vi "Event handler-Averages ValChange.vi"(11 "Averages.NewVal":u16) -> ()   [LabVIEW 2017]
uses:
  Global Variables/gl_UI Parameters.vi
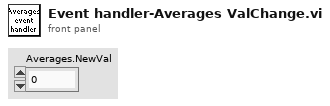
[diagram p1: front panel]
types:
  T1 = cluster{"Z Start":dbl, "Z Stop":dbl, "Z Step":dbl, "Pockels\n@Z Start":u8, "Pockels\n@Z Stop":u8, "# Planes":u16, "Dwell\nTime":sgl, "Zoom":i8, "# Averaged Frames":u16, "PMT 2":i16, "PMT 1":i16, "Laser":u8, "AOL Z":sgl, "Objective":string, "Frame Size":u16, "AOL Mode":u16, "Field of View":u16}
  T2 = typedef "AOL_Globals.ctl" = cluster{"Imaging Protocol":T3, "Number of POI":u16, "Number of Miniscans":u16, "Number of Trials":u16, "Number of Cycles ":u64, "# Averaged Frames":u16, "Laser power (%)":u8, "Pockels":dbl, "Acquisition Length (sec)":dbl, "Fill time (us)":dbl, "POI Dwell time (us)":dbl, "Miniscan Dwell time per pixel (us)":dbl, "PMT 1":dbl, "PMT 2":dbl, "Back Apperture":dbl, "Frame Size":T4, "Center Frequency":dbl, "Field of View":dbl, "DwellTime (us)":dbl, "Wavelength (nm)":dbl, "Zoom":dbl, "AOL Z":dbl, "AOL Mode":T5, "GridXY":dbl, "GridZ":dbl, "TriggerPeriod (sec)":dbl, "Number of Pixels in Miniscan":u16, "Experiment folder path":path, "X centre":dbl, "Y centre":dbl, "Angle (degrees)":dbl, "Plane Mode":T6, "Threshold":u16[], "Regenerate Chirps":bool, "Rectangle ROI length (pixels)":u16, "Rectangle ROI height (pixels)":u16, "AOD fill":u16, "StartupDelay":i32, "Samples Wait after Trigger":u16, "Slip Cycle":u32, "Add Cycle":bool}
  T3 = typedef "Imaging Protocols enum.ctl" = enum16{"AOL Z-Stack", "Motor Z Stack", "Functional Acquisition", "Single Plane Acquisition", "Volume Acquisition", "Live Imaging", "Live Plane Imaging", "Live Volume Imaging"}
  T4 = typedef "Frame Size.ctl" = u16
  T5 = typedef "AOL modes.ctl" = enum16{"Raster", "Structural", "Pointing", "Mini Scan", "Alignment"}
  T6 = typedef "Plane Mode.ctl" = u16
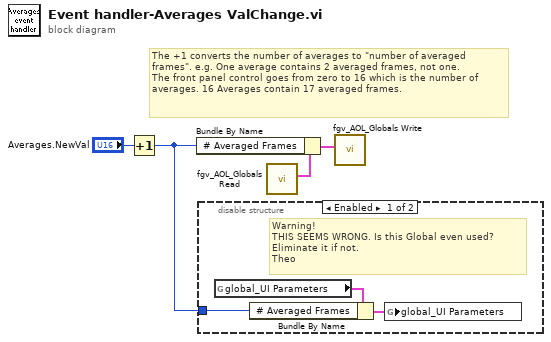
[diagram p0: block diagram]
diagram:
  # "The +1 converts the number of averages to \"number of averaged frames\". e.g. One average contains 2 averaged frames, not one.\nThe front panel control goes from zero to 16 which is the number of averages. 16 Averages contain 17 averaged frames."
  n1 = Increment(x="Averages.NewVal") -> (x+1=w4:u16)
  n2 = disable-structure shown="Enabled" {
    disable-tunnel: w4 -> [w5 _]
    frame Enabled {
      # "Warning!\nTHIS SEEMS WRONG. Is this Global even used? Eliminate it if not.\nTheo"
      n3 = global read "gl_UI Parameters.vi" "global_UI Parameters"() -> (w7:T1)
      n4 = Bundle By Name(cluster=w7, "# Averaged Frames"=w5) -> (w6:T1)
      n5 = global write "gl_UI Parameters.vi" "global_UI Parameters"(w6) -> ()
    }
    frame Disabled {
    }
  }
  n6 = call "fgv_AOL_Globals Read.vi"() -> ("AOL_Globals"=w2:T2)  [unwired: 9 in, 2 out]
  n7 = Bundle By Name(cluster=w2, "# Averaged Frames"=w4) -> (w1:T2)
  n8 = call "fgv_AOL_Globals Write.vi"("AOL_Globals"=w1) -> ()  [unwired: 10 in, 1 out]
